vi "ca.vi"(0 "IP adress":string="192.109.209.229", 1 "stop":bool, 2 "Channel":u8(ring) items=["1", "2", "3", "4", "5", "6", "7", "8", "9", "10", "11", "12", "13", "14", "15", "16"], 4 "Exit":bool, 5 "Start":bool, 6 "Draw":enum16{"Ewe(t)", "I(t)"}(ring)) -> (7 "XY Graph":cluster{"Data 101":sgl[], "Data 101":sgl[]}(graph)={"Data 101"=[0.0, 0.010008001, 0.020016002, 0.030024001, 0.040032003, 0.050040003, 0.060048003, 0.070056, 0.080064006, 0.090072006, 0.100080006, 0.110088006, 0.120096005, 0.130104, 0.140112, 0.15012, 0.16012801, 0.170136, 0.18014401, 0.190152, 0.20016001, 0.210168, 0.22017601, 0.230184, 0.24019201, 0.2502, 0.260208, 0.27021602, 0.280224, 0.290232, 0.30024, 0.31024802, 0.32025602, 0.330264, 0.340272, 0.35028002, 0.36028802, 0.370296, 0.380304, 0.39031202, 0.40032002, 0.410328, 0.420336, 0.43034402, 0.44035202, 0.45036003, 0.460368, 0.470376, 0.48038402, 0.49039203, 0.5004, 0.51040804, 0.520416, 0.530424, 0.54043204, 0.55044, 0.560448, 0.570456, 0.580464, 0.59047204, 0.60048, 0.610488, 0.62049603, 0.630504, 0.64051205, 0.65052, 0.660528, 0.67053604, 0.680544, 0.690552, 0.70056003, 0.710568, 0.72057605, 0.730584, 0.740592, 0.75060004, 0.760608, 0.77061605, 0.78062403, 0.790632, 0.80064005, 0.810648, 0.820656, 0.83066404, 0.840672, 0.85068005, 0.86068803, 0.870696, 0.88070405, 0.890712, 0.90072006, 0.91072804, 0.920736, 0.93074405, 0.940752, 0.95076, 0.96076804, 0.970776, 0.98078406, 0.99079204, 1.0008, 1.010808, 1.0208161, 1.0308241, 1.040832, 1.05084, 1.060848, 1.0708561, 1.0808641, 1.090872, 1.10088, 1.110888, 1.120896, 1.1309041, 1.140912, 1.15092, 1.160928, 1.170936, 1.1809441, 1.1909521, 1.20096, 1.210968, 1.220976, 1.2309841, 1.2409921, 1.251, 1.261008, 1.271016, 1.2810241, 1.2910321, 1.30104, 1.311048, 1.321056, 1.3310641, 1.3410721, 1.3510801, 1.361088, 1.371096, 1.381104, 1.3911121, 1.4011201, 1.411128, 1.421136, 1.431144, 1.4411521, 1.4511601, 1.461168, 1.471176, 1.481184, 1.4911921, 1.5012001, 1.511208, 1.521216, 1.531224, 1.5412321, 1.5512401, 1.5612481, 1.571256, 1.581264, 1.5912721, 1.6012801, 1.6112881, 1.621296, 1.631304, 1.641312, 1.6513201, 1.6613281, 1.671336, 1.681344, 1.691352, 1.7013601, 1.7113681, 1.7213761, 1.731384, 1.741392, 1.7514001, 1.7614081, 1.7714161, 1.781424, 1.791432, 1.8014401, 1.8114481, 1.8214561, 1.831464, 1.841472, 1.85148, 1.8614881, 1.8714961, 1.881504, 1.891512, 1.90152, 1.9115281, 1.9215361, 1.9315441, 1.941552, 1.95156, 1.9615681, 1.9715761, 1.9815841, 1.991592, 2.0016, 2.0116081, 2.021616, 2.031624, 2.0416322, 2.05164, 2.0616481, 2.071656, 2.081664, 2.0916722, 2.10168, 2.1116881, 2.121696, 2.131704, 2.1417122, 2.15172, 2.1617281, 2.171736, 2.181744, 2.1917522, 2.20176, 2.2117682, 2.221776, 2.231784, 2.241792, 2.2518, 2.2618082, 2.271816, 2.281824, 2.291832, 2.30184, 2.3118482, 2.321856, 2.331864, 2.341872, 2.35188, 2.3618882, 2.371896, 2.3819041, 2.391912, 2.40192, 2.4119282, 2.421936, 2.4319441, 2.441952, 2.45196, 2.4619682, 2.471976, 2.4819841, 2.491992, 2.502, 2.5120082, 2.522016, 2.5320241, 2.542032], "Data 101"=array[255 elements]}, 8 "Number of points":i32=255)   [LabVIEW 2016]
doc: "Chrono-Amperometry (CA) is a controlled-potential technique. The current response is measured to an applied potential step.\nIn general, in this VI, the first thing to do is to start by establishing the connection with the instrument defined by its IP adress, then load the firmware in the channel selected, get the information on the plugged channels, load protocol on a channel, start/stop the protocol, retreive data and draw the graph."
uses:
  LLB/dll_Functions.llb/CAParameters.ctl
panel:
  in  "Display Parameters?":bool caption="Display Parameters"
  out "DllPath":path caption="DLL Path"
  out "LibVersion":string caption="DLL Version"
  in  "CA Parameters":T1={"tb"=2.5e-05, "Steps"=[{"vs_initial"=TRUE, "Voltage_step"=0.0, "Duration_step"=1.0}, {"vs_initial"=TRUE, "Voltage_step"=0.1, "Duration_step"=1.0}, {"vs_initial"=TRUE, "Voltage_step"=0.2, "Duration_step"=1.0}], "Step_number"=2, "N_Cycles"=0, "Record_every_dI"=1e-05, "Record_every_dT"=0.01, "I_Range"=8, "E_Range"=3, "Bandwidth"=5, "em"=1, "ce"=0} {"tb" min=2.5e-05 max=1 format="%^_3e"; "ce" items=["Standard", "CE to ground"]; "N_Cycles" min=0 max=1000000; "Step_number" min=0 max=99; "E_Range" items=["±2.5V", "±5V", "±10V", "Auto"]; "Bandwidth" items=["1"=1, "2"=2, "3"=3, "4"=4, "5"=5, "6"=6, "7"=7, "8"=8, "9"=9]; "Record_every_dT" min=0.0001 max=1000 format="%^_3e"; "Record_every_dI" format="%^_3e"; "I_Range" items=["1pA", "1nA", "10nA", "100nA", "1µA", "10µA", "100µA", "1mA", "10mA", "100mA", "1A", "Booster", "Auto"]; "Steps"."Duration_step" min=0.001 max=80000 format="%^_3e"; "Steps"."Voltage_step" min=-10 max=10 format="%^_3e"}
  out "Exit 2":bool=TRUE
  out "Data 101":sgl[][](array[numeric])=[[0.0, -0.00011507986, 2.9229916e-06, 1.0], [0.010008001, -0.00048330438, 2.9229916e-06, 1.0], [0.020016002, -0.00048330438, 2.9229916e-06, 1.0], [0.030024001, -0.0007121685, 6.7342776e-06, 1.0], [0.040032003, -0.0007121685, 3.6852487e-06, 1.0], [0.050040003, -0.00063588045, 6.362202e-07, 1.0], [0.060048003, -0.00048330438, 5.2097635e-06, 1.0], [0.070056, -0.0004070163, 2.1607345e-06, 1.0], [0.080064006, -0.00017815214, 3.6852487e-06, 1.0], [0.090072006, -0.0004070163, 3.6852487e-06, 1.0], [0.100080006, -0.0004070163, 2.1607345e-06, 1.0], [0.110088006, -0.00063588045, 2.9229916e-06, 1.0], [0.120096005, -0.0005595924, 2.9229916e-06, 1.0], [0.130104, -0.0007121685, 5.2097635e-06, 1.0], [0.140112, -0.00033072825, 5.2097635e-06, 1.0], [0.15012, -0.00063588045, 2.9229916e-06, 1.0], [0.16012801, -0.0007884566, 1.3984774e-06, 1.0], [0.170136, -0.0004070163, 5.2097635e-06, 1.0], [0.18014401, -0.00063588045, 3.6852487e-06, 1.0], [0.190152, -0.00063588045, 5.97202e-06, 1.0], [0.20016001, -0.0007121685, 5.2097635e-06, 1.0], [0.210168, -0.00033072825, 2.9229916e-06, 1.0], [0.22017601, -0.0007121685, 1.3984774e-06, 1.0], [0.230184, -0.00063588045, 5.97202e-06, 1.0], [0.24019201, -0.0007884566, 5.97202e-06, 1.0], [0.2502, -0.00063588045, 4.447506e-06, 1.0], [0.260208, -0.00063588045, 4.447506e-06, 1.0], [0.27021602, -0.0007884566, 3.6852487e-06, 1.0], [0.280224, -0.00025444018, 2.9229916e-06, 1.0], [0.290232, -0.00063588045, 4.447506e-06, 1.0], [0.30024, -0.0007884566, 5.2097635e-06, 1.0], [0.31024802, -0.00048330438, 2.9229916e-06, 1.0], [0.32025602, -0.00063588045, 2.1607345e-06, 1.0], [0.330264, -0.00063588045, 3.6852487e-06, 1.0], [0.340272, -0.00063588045, 2.9229916e-06, 1.0], [0.35028002, -0.00017815214, 5.2097635e-06, 1.0], [0.36028802, -0.0007884566, 5.97202e-06, 1.0], [0.370296, -0.00063588045, 2.9229916e-06, 1.0], [0.380304, -0.00086474465, 6.7342776e-06, 1.0], [0.39031202, -0.0004070163, 2.9229916e-06, 1.0], [0.40032002, -0.0007884566, 6.362202e-07, 1.0], [0.410328, -0.0007121685, 2.1607345e-06, 1.0], [0.420336, -0.0007884566, 6.7342776e-06, 1.0], [0.43034402, -0.00063588045, 1.3984774e-06, 1.0], [0.44035202, -0.00063588045, 2.9229916e-06, 1.0], [0.45036003, -0.00063588045, 2.1607345e-06, 1.0], [0.460368, -0.00048330438, 4.447506e-06, 1.0], [0.470376, -0.00048330438, 4.447506e-06, 1.0], [0.48038402, -0.0004070163, 2.9229916e-06, 1.0], [0.49039203, -0.00033072825, 5.2097635e-06, 1.0], [0.5004, -0.00048330438, 5.2097635e-06, 1.0], [0.51040804, -0.0005595924, 5.2097635e-06, 1.0], [0.520416, -0.0005595924, 5.97202e-06, 1.0], [0.530424, -0.0007121685, 5.2097635e-06, 1.0], [0.54043204, -0.0004070163, 2.9229916e-06, 1.0], [0.55044, -0.00025444018, 5.2097635e-06, 1.0], [0.560448, -0.00048330438, 2.9229916e-06, 1.0], [0.570456, -0.0004070163, 4.447506e-06, 1.0], [0.580464, -0.0004070163, 2.9229916e-06, 1.0], [0.59047204, -0.00063588045, 2.1607345e-06, 1.0], [0.60048, -0.0007884566, 2.1607345e-06, 1.0], [0.610488, -0.00048330438, 5.2097635e-06, 1.0], [0.62049603, -0.0004070163, 2.9229916e-06, 1.0], [0.630504, -0.0007884566, 3.6852487e-06, 1.0], [0.64051205, -0.0007884566, 2.9229916e-06, 1.0], [0.65052, -0.0005595924, 5.97202e-06, 1.0], [0.660528, -0.00048330438, 2.9229916e-06, 1.0], [0.67053604, -0.00063588045, 4.447506e-06, 1.0], [0.680544, -0.00086474465, 4.447506e-06, 1.0], [0.690552, -0.00063588045, 3.6852487e-06, 1.0], [0.70056003, -0.00063588045, 1.3984774e-06, 1.0], [0.710568, -0.0005595924, 4.447506e-06, 1.0], [0.72057605, -0.00048330438, 2.9229916e-06, 1.0], [0.730584, -0.00048330438, 3.6852487e-06, 1.0], [0.740592, -0.0007884566, 4.447506e-06, 1.0], [0.75060004, -0.0005595924, 3.6852487e-06, 1.0], [0.760608, -0.0005595924, 2.9229916e-06, 1.0], [0.77061605, -0.0007884566, 4.447506e-06, 1.0], [0.78062403, -0.0010173208, 2.1607345e-06, 1.0], [0.790632, -0.00063588045, 2.1607345e-06, 1.0], [0.80064005, -0.00025444018, 2.9229916e-06, 1.0], [0.810648, -0.0005595924, 3.6852487e-06, 1.0], [0.820656, -0.00017815214, 3.6852487e-06, 1.0], [0.83066404, -0.0005595924, 4.447506e-06, 1.0], [0.840672, -0.0005595924, 1.3984774e-06, 1.0], [0.85068005, -0.00063588045, 5.2097635e-06, 1.0], [0.86068803, -0.0007884566, 5.97202e-06, 1.0], [0.870696, -0.0004070163, 4.447506e-06, 1.0], [0.88070405, -0.00033072825, 4.447506e-06, 1.0], [0.890712, -0.0005595924, 3.6852487e-06, 1.0], [0.90072006, -0.0005595924, 4.447506e-06, 1.0], [0.91072804, -0.0007121685, 4.447506e-06, 1.0], [0.920736, -0.00063588045, 2.1607345e-06, 1.0], [0.93074405, -0.0005595924, 5.2097635e-06, 1.0], [0.940752, -0.0004070163, 2.1607345e-06, 1.0], [0.95076, -0.0004070163, 2.1607345e-06, 1.0], [0.96076804, -0.00025444018, 2.9229916e-06, 1.0], [0.970776, -0.00063588045, 3.6852487e-06, 1.0], [0.98078406, -0.00063588045, 2.9229916e-06, 1.0], [0.99079204, 0.0001270001, 2.1607345e-06, 1.0], [1.0008, 0.09945406, 5.5518736e-05, 1.0], [1.010808, 0.09960663, 2.3503935e-05, 1.0], [1.0208161, 0.09945406, 2.2741679e-05, 1.0], [1.0308241, 0.099759206, 2.5790707e-05, 1.0], [1.040832, 0.09930148, 2.4266194e-05, 1.0], [1.05084, 0.099377766, 2.1217164e-05, 1.0], [1.060848, 0.09945406, 2.2741679e-05, 1.0], [1.0708561, 0.09953035, 2.1217164e-05, 1.0], [1.0808641, 0.09953035, 2.3503935e-05, 1.0], [1.090872, 0.09953035, 2.3503935e-05, 1.0], [1.10088, 0.09968292, 2.4266194e-05, 1.0], [1.110888, 0.09945406, 2.4266194e-05, 1.0], [1.120896, 0.09953035, 2.6552963e-05, 1.0], [1.1309041, 0.099377766, 2.6552963e-05, 1.0], [1.140912, 0.09953035, 2.502845e-05, 1.0], [1.15092, 0.09922519, 2.1217164e-05, 1.0], [1.160928, 0.09953035, 2.3503935e-05, 1.0], [1.170936, 0.099377766, 1.969265e-05, 1.0], [1.1809441, 0.09930148, 2.4266194e-05, 1.0], [1.1909521, 0.09953035, 2.4266194e-05, 1.0], [1.20096, 0.09953035, 2.3503935e-05, 1.0], [1.210968, 0.09953035, 2.4266194e-05, 1.0], [1.220976, 0.09968292, 2.2741679e-05, 1.0], [1.2309841, 0.09960663, 2.4266194e-05, 1.0], [1.2409921, 0.0998355, 2.4266194e-05, 1.0], [1.251, 0.09945406, 2.1217164e-05, 1.0], [1.261008, 0.09968292, 2.502845e-05, 1.0], [1.271016, 0.09930148, 2.4266194e-05, 1.0], [1.2810241, 0.09968292, 1.8930392e-05, 1.0], [1.2910321, 0.09930148, 2.4266194e-05, 1.0], [1.30104, 0.09930148, 2.5790707e-05, 1.0], [1.311048, 0.09907261, 2.4266194e-05, 1.0], [1.321056, 0.09945406, 2.1217164e-05, 1.0], [1.3310641, 0.09968292, 2.5790707e-05, 1.0], [1.3410721, 0.09914891, 2.1979422e-05, 1.0], [1.3510801, 0.09945406, 2.502845e-05, 1.0], [1.361088, 0.09945406, 2.5790707e-05, 1.0], [1.371096, 0.09960663, 2.1217164e-05, 1.0], [1.381104, 0.09930148, 2.4266194e-05, 1.0], [1.3911121, 0.09930148, 2.4266194e-05, 1.0], [1.4011201, 0.09998807, 2.4266194e-05, 1.0], [1.411128, 0.09968292, 2.4266194e-05, 1.0], [1.421136, 0.09960663, 2.1217164e-05, 1.0], [1.431144, 0.09998807, 2.3503935e-05, 1.0], [1.4411521, 0.09968292, 2.1217164e-05, 1.0], [1.4511601, 0.09953035, 2.5790707e-05, 1.0], [1.461168, 0.09960663, 2.5790707e-05, 1.0], [1.471176, 0.09968292, 2.2741679e-05, 1.0], [1.481184, 0.09930148, 2.4266194e-05, 1.0], [1.4911921, 0.09945406, 2.2741679e-05, 1.0], [1.5012001, 0.09960663, 2.0454907e-05, 1.0], [1.511208, 0.09945406, 2.3503935e-05, 1.0], [1.521216, 0.099377766, 1.969265e-05, 1.0], [1.531224, 0.09930148, 2.1217164e-05, 1.0], [1.5412321, 0.09914891, 2.2741679e-05, 1.0], [1.5512401, 0.09953035, 2.2741679e-05, 1.0], [1.5612481, 0.099377766, 2.2741679e-05, 1.0], [1.571256, 0.099377766, 2.5790707e-05, 1.0], [1.581264, 0.099759206, 2.4266194e-05, 1.0], [1.5912721, 0.09968292, 2.2741679e-05, 1.0], [1.6012801, 0.09930148, 2.4266194e-05, 1.0], [1.6112881, 0.09930148, 2.4266194e-05, 1.0], [1.621296, 0.09960663, 2.1217164e-05, 1.0], [1.631304, 0.09968292, 2.5790707e-05, 1.0], [1.641312, 0.09953035, 2.5790707e-05, 1.0], [1.6513201, 0.09930148, 2.502845e-05, 1.0], [1.6613281, 0.09945406, 2.4266194e-05, 1.0], [1.671336, 0.09953035, 2.1217164e-05, 1.0], [1.681344, 0.099377766, 2.4266194e-05, 1.0], [1.691352, 0.09960663, 2.2741679e-05, 1.0], [1.7013601, 0.09968292, 2.3503935e-05, 1.0], [1.7113681, 0.09907261, 2.5790707e-05, 1.0], [1.7213761, 0.09953035, 2.4266194e-05, 1.0], [1.731384, 0.099377766, 2.2741679e-05, 1.0], [1.741392, 0.09960663, 2.502845e-05, 1.0], [1.7514001, 0.09953035, 2.502845e-05, 1.0], [1.7614081, 0.09945406, 2.6552963e-05, 1.0], [1.7714161, 0.099377766, 2.502845e-05, 1.0], [1.781424, 0.09960663, 2.5790707e-05, 1.0], [1.791432, 0.09907261, 2.502845e-05, 1.0], [1.8014401, 0.09930148, 2.0454907e-05, 1.0], [1.8114481, 0.09968292, 2.1979422e-05, 1.0], [1.8214561, 0.09930148, 2.2741679e-05, 1.0], [1.831464, 0.09930148, 2.4266194e-05, 1.0], [1.841472, 0.09914891, 2.0454907e-05, 1.0], [1.85148, 0.099377766, 2.2741679e-05, 1.0], [1.8614881, 0.09953035, 2.502845e-05, 1.0], [1.8714961, 0.09945406, 2.3503935e-05, 1.0], [1.881504, 0.09907261, 2.502845e-05, 1.0], [1.891512, 0.099377766, 2.2741679e-05, 1.0], [1.90152, 0.09945406, 2.5790707e-05, 1.0], [1.9115281, 0.09953035, 2.5790707e-05, 1.0], [1.9215361, 0.099759206, 2.4266194e-05, 1.0], [1.9315441, 0.09945406, 2.6552963e-05, 1.0], [1.941552, 0.09945406, 2.0454907e-05, 1.0], [1.95156, 0.09945406, 2.5790707e-05, 1.0], [1.9615681, 0.09991179, 2.5790707e-05, 1.0], [1.9715761, 0.09945406, 2.3503935e-05, 1.0], [1.9815841, 0.09930148, 2.3503935e-05, 1.0], [1.991592, 0.09960663, 2.5790707e-05, 1.0], [2.0016, 0.19969657, 6.3903564e-05, 1.0], [2.0116081, 0.19939142, 4.256037e-05, 1.0], [2.021616, 0.19931513, 4.408488e-05, 1.0], [2.031624, 0.1994677, 4.332262e-05, 1.0], [2.0416322, 0.199544, 4.332262e-05, 1.0], [2.05164, 0.1994677, 4.4847136e-05, 1.0], [2.0616481, 0.19962028, 4.332262e-05, 1.0], [2.071656, 0.19977286, 4.332262e-05, 1.0], [2.081664, 0.19992544, 4.256037e-05, 1.0], [2.0916722, 0.19977286, 4.4847136e-05, 1.0], [2.10168, 0.19977286, 4.408488e-05, 1.0], [2.1116881, 0.20007801, 4.4847136e-05, 1.0], [2.121696, 0.19992544, 4.103585e-05, 1.0], [2.131704, 0.199544, 4.256037e-05, 1.0], [2.1417122, 0.199544, 4.6371653e-05, 1.0], [2.15172, 0.19969657, 4.256037e-05, 1.0], [2.1617281, 0.199544, 4.256037e-05, 1.0], [2.171736, 0.19984914, 4.256037e-05, 1.0], [2.181744, 0.1994677, 4.256037e-05, 1.0], [2.1917522, 0.20000172, 4.256037e-05, 1.0], [2.20176, 0.199544, 4.6371653e-05, 1.0], [2.2117682, 0.1994677, 4.0273593e-05, 1.0], [2.221776, 0.19969657, 4.332262e-05, 1.0], [2.231784, 0.19962028, 4.332262e-05, 1.0], [2.241792, 0.199544, 4.408488e-05, 1.0], [2.2518, 0.19977286, 4.332262e-05, 1.0], [2.2618082, 0.1994677, 4.408488e-05, 1.0], [2.271816, 0.19969657, 4.6371653e-05, 1.0], [2.281824, 0.19969657, 4.408488e-05, 1.0], [2.291832, 0.1994677, 4.332262e-05, 1.0], [2.30184, 0.19984914, 4.408488e-05, 1.0], [2.3118482, 0.19923884, 3.9511335e-05, 1.0], [2.321856, 0.19962028, 4.256037e-05, 1.0], [2.331864, 0.19969657, 4.1798106e-05, 1.0], [2.341872, 0.19969657, 4.6371653e-05, 1.0], [2.35188, 0.19969657, 4.4847136e-05, 1.0], [2.3618882, 0.19969657, 4.6371653e-05, 1.0], [2.371896, 0.19939142, 4.103585e-05, 1.0], [2.3819041, 0.19939142, 4.332262e-05, 1.0], [2.391912, 0.1994677, 4.103585e-05, 1.0], [2.40192, 0.19962028, 4.1798106e-05, 1.0], [2.4119282, 0.19962028, 4.4847136e-05, 1.0], [2.421936, 0.1994677, 4.332262e-05, 1.0], [2.4319441, 0.19977286, 4.408488e-05, 1.0], [2.441952, 0.20007801, 4.408488e-05, 1.0], [2.45196, 0.19984914, 4.5609395e-05, 1.0], [2.4619682, 0.19962028, 4.256037e-05, 1.0], [2.471976, 0.19984914, 4.4847136e-05, 1.0], [2.4819841, 0.19939142, 4.6371653e-05, 1.0], [2.491992, 0.199544, 4.1798106e-05, 1.0], [2.502, 0.19984914, 4.408488e-05, 1.0], [2.5120082, 0.19931513, 4.332262e-05, 1.0], [2.522016, 0.199544, 4.6371653e-05, 1.0], [2.5320241, 0.199544, 4.4847136e-05, 1.0], [2.542032, 0.19931513, 4.408488e-05, 1.0]] format="%.2f"
  # "Instructions:\nBefore running the VI you must type a valid IP adress that corresponds to the instrument.Then press the Run button to execute this VI.\nWhile this VI is running, choose the available channel, enter the CA parameters or keep the default values, then press the start button to begin the experience.\nChoose the waveform to draw (Ewe(t) or I(t)). You can stop the measure if you press the stop button and exit the execution if you press the exit button."
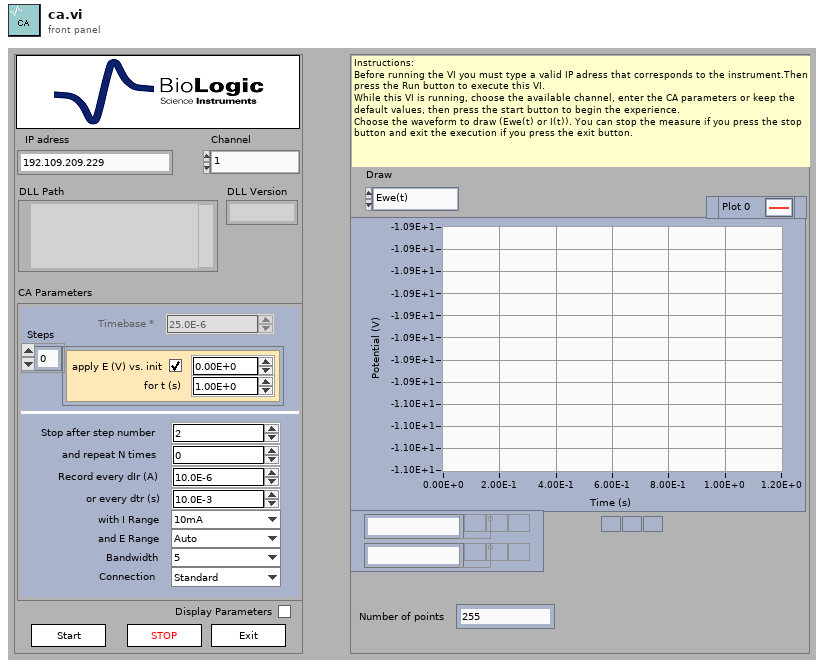
[diagram p1: front panel]
types:
  T1 = typedef "CAParameters.ctl" = cluster{"tb":sgl, "Steps":cluster{"vs_initial":bool, "Voltage_step":sgl, "Duration_step":sgl}[], "Step_number":i32, "N_Cycles":i32, "Record_every_dI":sgl, "Record_every_dT":sgl, "I_Range":u16, "E_Range":u16, "Bandwidth":u16, "em":u16, "ce":u16}
  T2 = cluster{"LibVersion":string, "StringLength":u32, "DllPath":path}
  T3 = cluster{"Channel":i32, "BoardVersion":i32, "BoardSerialCode":i32, "FirmwareCode":i32, "FirmwareVersion":i32, "XilinxVersion":i32, "AmpCode":i32, "NbAmp":i32, "LcBoard":i32, "Zboard":i32, "MuxBoard":i32, "GPRAboard":i32, "MemSize":i32, "MemFilled":i32, "state":i32, "MaxIRange":i32, "MinIRange":i32, "MaxBandwidth":i32, "NbOfTechniques":i32}
  T4 = typedef "TechniqueParameters.ctl" = cluster{"String Label":string, "Type":i32, "Valeur":i32, "Index":i32}
  T5 = cluster{"string before end tag":string, i32, i32, i32}[]
  T6 = cluster{"IRQskipped":i32, "NbRaws":i32, "NbCols":i32, "Technique Index":i32, "TechniqueID":i32, "PrcessIndex":i32, "loop":i32, "StartTime":dbl, "MuxPad":i32}
  T7 = cluster{"State":i32, "MemFilled":i32, "TimeBase":sgl, " Ewe":sgl, " EweRangeMin":sgl, " EweRangeMax":sgl, "Ece":sgl, "EceRangeMin":sgl, "EceRangeMax":sgl, "Eoverflow":i32, "I":sgl, "IRange":i32, "Ioverflow":i32, "ElapsedTime":sgl, "Freq":sgl, "Rcomp":sgl, "Saturation":sgl, "OptErr":i32, "OptPos":i32}
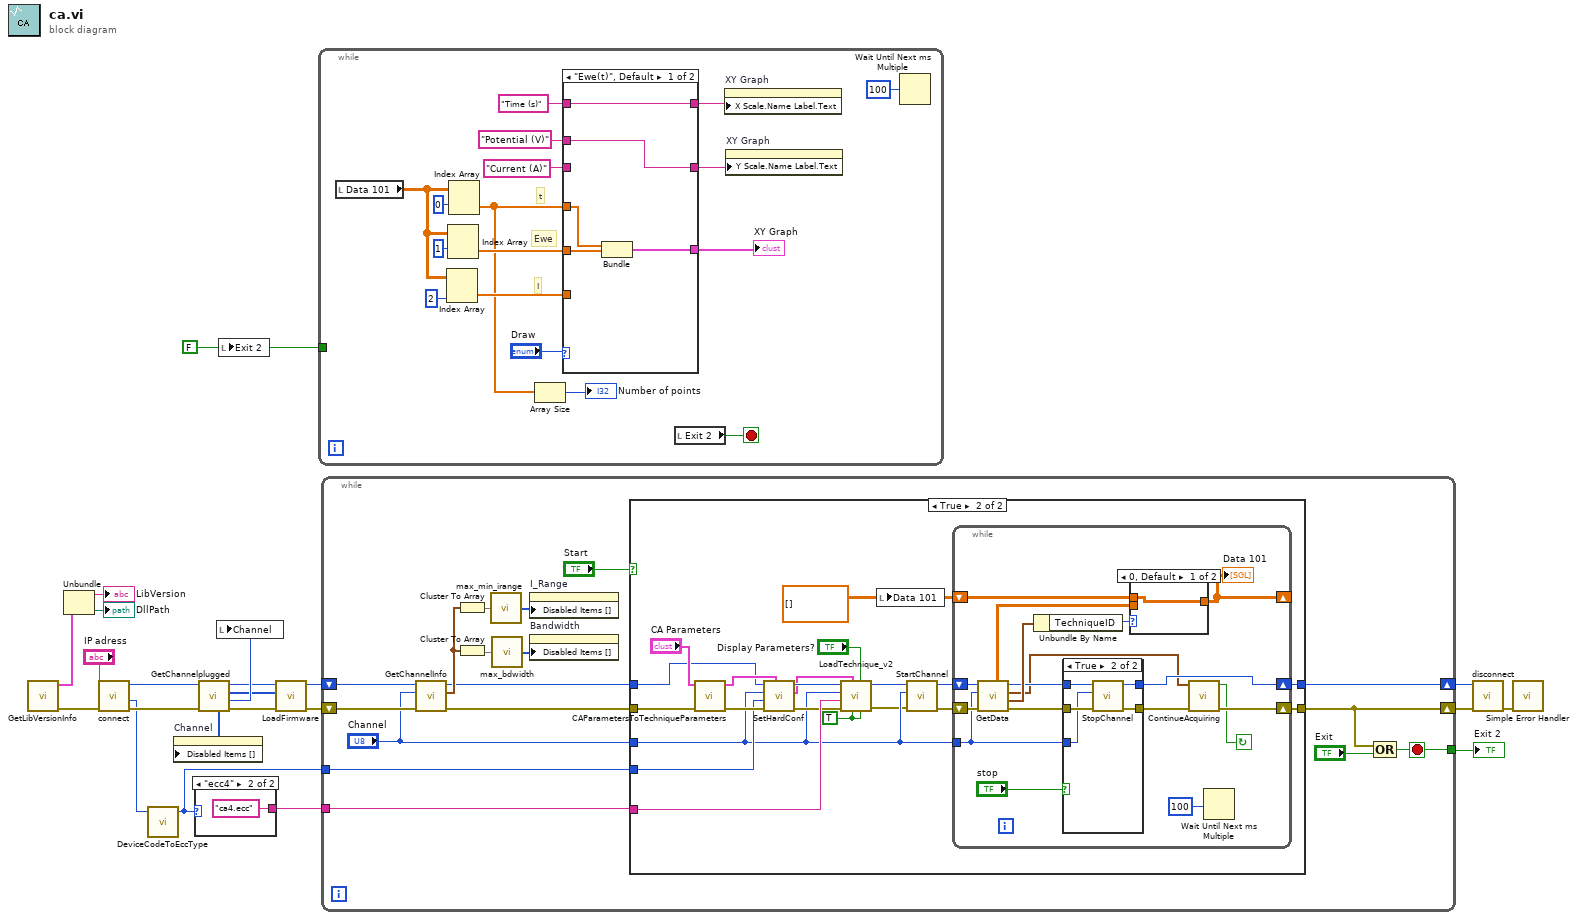
[diagram p0: block diagram]
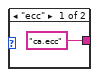
[diagram p2: hidden frame]
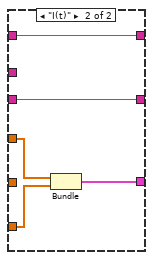
[diagram p3: hidden frame]
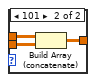
[diagram p6: hidden frame]
diagram:
  w21 = FALSE ("Exit 2")
  n1 = call "GetLibVersionInfo.vi"() -> ("error out"=w4:errorcluster, "LibInfo"=w3:T2)  [unwired: 10 in]
  n2 = Unbundle(w3) -> ("LibVersion"=→"LibVersion":string, "DllPath"=→"DllPath":path)  [unwired: 1 out]
  n3 = call "connect.vi"("error in (no error)"=w4, "IP"="IP adress") -> ("error out"=w17:errorcluster, "Device Code"=w6:i32, "ID Out"=w13:i32)  [unwired: 6 in, 1 out]
  n4 = call "DeviceCodeToEccType.vi"("Device Code"=w6) -> ("EccType"=w5:enum16{"ecc", "ecc4"})  [unwired: 4 in]
  n5 = case shown="\"ecc4\"" w5 {
    tunnel: ["ca.ecc" ("FName") "ca4.ecc" ("FName")] -> w8
    frame "ecc" {
    }
    frame "ecc4" {
    }
  }
  n6 = call "GetChannelplugged.vi"("error in (no error)"=w17, "ID In"=w13) -> ("error out"=w16:errorcluster, "FirstPluggedChannel"=w19:u8, "PluggedChannels"=w14:u8[], "ID Out"=w12:i32, "DisabledChannels"=w15:i32[])  [unwired: 5 in]
  n7 = property on="Channel" class="Ring (strict)"("Disabled Items []"=w15) -> ()  [unwired: 2 in, 2 out]
  n8 = local write "Channel"(w19) -> ()
  n9 = local write "Exit 2"(w21) -> ()
  n10 = call "LoadFirmware.vi"("error in (no error)"=w16, "Channels"=w14, "ID In"=w12) -> ("error out"=w11:errorcluster, "ID Out"=w10:i32)  [unwired: 6 in, 1 out]
  n11 = while {
    tunnel: w21 -> [_]
    stop <- w40 stop-if-true
    # "I"
    # "Ewe"
    # "t"
    n12 = local read "Data 101"() -> (w29:sgl[][])
    n13 = Index Array(array=w29, index (col)=2 ("indice désactivé (col)")) -> (element=w26:sgl[])  [unwired: 1 in]
    n14 = Index Array(array=w29, index (col)=1 ("Index")) -> (element=w28:sgl[])  [unwired: 1 in]
    n15 = Index Array(array=w29, index (col)=0 ("Index")) -> (element=w25:sgl[])  [unwired: 1 in]
    n16 = Array Size(array=w25) -> (size(s)=→"Number of points":i32)
    n17 = case shown="\"Ewe(t)\", Default" "Draw" {
      tunnel: w25 -> [w46 w47]
      tunnel: [w43 w48] -> w27
      tunnel: "Potential (V)" ("Y Scale.Name Label.Text") -> [w45 _]
      tunnel: "Current (A)" ("Y Scale.Name Label.Text") -> [_ w51]
      tunnel: [w45 w51] -> w34
      tunnel: [w44 w50] -> w33
      tunnel: "Time (s)" ("Y Scale.Name Label.Text") -> [w44 w50]
      tunnel: w28 -> [w42 _]
      tunnel: w26 -> [_ w49]
      frame "Ewe(t)", Default {
        n18 = Bundle("Data 101"=w46, "Data 101"=w42) -> (w43:cluster{"Data 101":sgl[], "Data 101":sgl[]})  [unwired: 1 in]
      }
      frame "I(t)" {
        n19 = Bundle("Data 101"=w47, "Data 101"=w49) -> (w48:cluster{"Data 101":sgl[], "Data 101":sgl[]})  [unwired: 1 in]
      }
    }
    "XY Graph" <- w27
    n20 = local read "Exit 2"() -> (w40:bool)
    n21 = property on="XY Graph" class="XYGraph (strict)"("X Scale.Name Label.Text"=w33) -> ()  [unwired: 2 in, 2 out]
    n22 = property on="XY Graph" class="XYGraph (strict)"("Y Scale.Name Label.Text"=w34) -> ()  [unwired: 2 in, 2 out]
    n23 = Wait Until Next ms Multiple(millisecond multiple=u32 100) -> ()  [unwired: 1 out]
  }
  n24 = while {
    shift-right: [w55] -> w9
    shift-left: w11 -> [w61]
    tunnel: [w53] -> w22
    shift-right: [w65] -> w18
    shift-left: w10 -> [w62]
    tunnel: w8 -> [w56]
    tunnel: w5 -> [w52]
    stop <- w53 stop-if-true
    n25 = call "GetChannelInfo.vi"("error in (no error)"=w61, "Channel"="Channel", "ID"=w62) -> ("error out"=w59:errorcluster, "Channel information"=w60:T3, "ID Out"=w58:i32)  [unwired: 6 in]
    n26 = Cluster To Array(cluster=w60) -> (array=w67:i32[])
    n27 = Cluster To Array(cluster=w60) -> (array=w66:i32[])
    n28 = call "max_min_irange.vi"("resources"=w67) -> ("disabled ranges"=w63:i32[])
    n29 = call "max_bdwidth.vi"("resources"=w66) -> ("disabled ranges"=w64:i32[])
    n30 = property on="I_Range" class="Ring (strict)"("Disabled Items []"=w63) -> ()  [unwired: 2 in, 2 out]
    n31 = property on="Bandwidth" class="Ring (strict)"("Disabled Items []"=w64) -> ()  [unwired: 2 in, 2 out]
    n32 = case shown="True" "Start" {
      tunnel: "Channel" -> [_ w74]
      tunnel: [w70 w84] -> w55
      tunnel: w59 -> [w70 w83]
      tunnel: w58 -> [w69 w75]
      tunnel: [w69 w85] -> w65
      tunnel: w56 -> [_ w88]
      tunnel: w52 -> [_ w76]
      frame False {
      }
      frame True {
        w87 = TRUE ("First Protocol")
        w90 = sgl[][] []
        n33 = call "CAParametersToTechniqueParameters.vi"("error in (no error)"=w83, "CA Parameters"="CA Parameters") -> ("error out"=w82:errorcluster, "Params Values"=w79:T4[])  [unwired: 8 in]
        n34 = call "SetHardConf.vi"("Params Values"=w79, "error in (no error)"=w82, "EccType"=w76, "Channel"=w74, "ID In"=w75) -> ("error out"=w77:errorcluster, "Params Values Trimed"=w78:T5, "ID Out"=w81:i32)  [unwired: 4 in]
        n35 = call "LoadTechnique_v2.vi"("Last Protocol"=w87, "Display Parameters?"="Display Parameters?", "First Protocol"=w87, "TechniqueParameters"=w78, "error in (no error)"=w77, "FName"=w88, "Selected Channel"=w74, "ID In"=w81) -> ("error out"=w73:errorcluster, "ID  Out"=w72:i32)  [unwired: 2 in]
        n36 = local write "Data 101"(w90) -> ()
        n37 = call "StartChannel.vi"("error in (no error)"=w73, "Channel"=w74, "ID In"=w72) -> ("error out"=w89:errorcluster, "ID Out"=w86:i32)  [unwired: 7 in]
        n38 = while {
          shift-right: [w94] -> w84
          shift-left: w89 -> [w107]
          shift-right: [w104] -> _
          shift-left: w90 -> [w105]
          tunnel: w74 -> [w102]
          shift-right: [w96] -> w85
          shift-left: w86 -> [w98]
          stop <- w91 continue-if-true
          n39 = call "GetData.vi"("error in (no error)"=w107, "Channel"=w102, "ID In"=w98) -> ("error out"=w95:errorcluster, "Data information"=w101:T6, "Current values"=w92:T7, "ID Out"=w97:i32, "Data"=w99:dbl[][])  [unwired: 4 in]
          n40 = Unbundle By Name(w101) -> ("TechniqueID"=w100:i32)
          n41 = case shown="True" "stop" {
            tunnel: [w109 w114] -> w93
            tunnel: w95 -> [w109 w113]
            tunnel: w102 -> [_ w112]
            tunnel: w97 -> [w108 w111]
            tunnel: [w108 w110] -> w96
            frame False {
            }
            frame True {
              n42 = call "StopChannel.vi"("error in (no error)"=w113, "Channel"=w112, "ID In"=w111) -> ("error out"=w114:errorcluster, "ID Out"=w110:i32)  [unwired: 7 in]
            }
          }
          n43 = case shown="0, Default" w100 {
            tunnel: w99 -> [_ w118]
            tunnel: w105 -> [w115 w117]
            tunnel: [w115 w116] -> w104
            frame 0, Default {
            }
            frame 101 {
              n44 = Build Array (concatenate)(w117, w118) -> (w116:dbl[][])
            }
          }
          "Data 101" <- w104
          n45 = call "ContinueAcquiring.vi"("error in"=w93, "Current values"=w92) -> ("error out"=w94:errorcluster, "ContinueAcquiring?"=w91:bool)  [unwired: 8 in]
          n46 = Wait Until Next ms Multiple(millisecond multiple=u32 100) -> ()  [unwired: 1 out]
        }
      }
    }
    n47 = Compound Arithmetic op=OR(w55, "Exit") -> (w53:bool)
  }
  "Exit 2" <- w22
  n48 = call "disconnect.vi"("error in (no error)"=w9, "ID In"=w18) -> ("error out"=w7:errorcluster)  [unwired: 9 in]
  n49 = call <vilib>:"Simple Error Handler.vi"("error in (no error)"=w7) -> ()  [unwired: 4 in, 5 out]
